vi "AuMT8852B Boolean Attribute.vi"(5 "Value (F)":bool, 7 "Set/Get (Set)":enum16{"Set", "Get"}(ring), 8 "error in (no error)":errorcluster, 10 "Attribute ID":T3, 11 "VISA session":refnum<visa-resource-name>) -> (0 "error out":errorcluster, 3 "VISA session out":refnum<visa-resource-name>, 4 "Value out":bool, 6 "Status":T1=enum."I/O needed")   [LabVIEW 2017]
doc: "Anritsu MT8852B Bluetooth Tester\n\nReconciles attribute values with the cached copies.\n\nINPUTS\nSet/Get - whether the value is being written or read.\nAttribute ID - which value is being written or read.\nValue - attribute to write.\n\nOUTPUTS\nStatus - Instrument I/O will be necessary if simulation is on, caching is off, or caching is on but the cached value is different or invalid.\nValue out - value from the cache."
uses:
  <instrlib>/aumt8852B/General/Utilities/MT8850 Attribute ID.ctl
  <instrlib>/aumt8852B/General/Utilities/Instrument.llb/Instrument Object Reference.ctl
  <instrlib>/aumt8852B/General/Utilities/Instrument.llb/Attribute Status.ctl
panel:
  in  "reference":T2
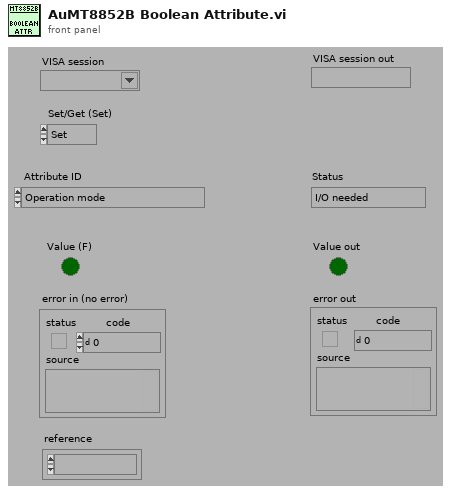
[diagram p1: front panel]
types:
  T1 = typedef "Attribute Status.ctl" = enum16{"No I/O needed", "I/O needed"}
  T2 = typedef "Instrument Object Reference.ctl" = refnum<k1>
  T3 = typedef "MT8850 Attribute ID.ctl" = enum16{"Operation mode", "Selected script", "EUT address source", "EUT Address", "EUT HCI RS232 Baud Rate", "Tester GPIB Address", "Tester RS232 Baud Rate", "Tester Bluetooth Address", "Tester Contrast", "Tester Key Click On", "Tester Modulation Index", "Tester Poll-Null Mode", "Tester Power Range", "Tester RS232 Mode", "Beep on Illegal Entry", "Display User Text", "User Text", "Calibration TX Modulation DAC", "Calibration RX Channel", "Calibration TX Channel", "Calibration TX Power", "Calibration Use TX Table", "Inquiry Request User-friendly Name", "Inquiry Number of Responses", "Inquiry Timeout", "Script Frequency Display", "Script Loop Count", "Script Loop Continuously", "Script Loop Stop on Fail", "Link timeout", "Page timeout", "Filter bandwidth", "SCO air code", "SCO bit position", "SCO input code", "SCO input data", "SCO input sample size", "SCO loopback mode", "SCO packet type", "SCO tone generator", "Tester page scan repetition mode", "Tester follow test mode", "Tester authentication state", "Tester authentication pin code", "Tester authentication pin length"}
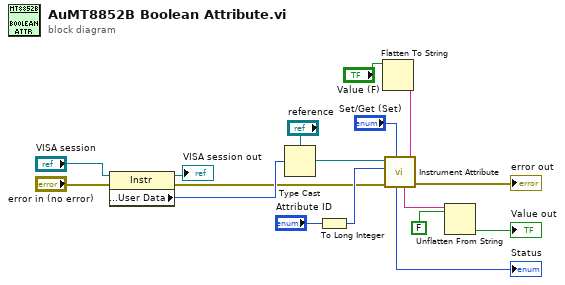
[diagram p0: block diagram]
diagram:
  n1 = property class="Instr"(reference="VISA session", error in="error in (no error)") -> (reference out=→"VISA session out":refnum<visa-resource-name>, error out=w5:errorcluster, "General Settings:User Data"=w11:u32)
  n2 = Type Cast(type="reference", x=w11) -> (*(type *) &x=w9:T2)
  n3 = To Long Integer(number="Attribute ID") -> (32bit integer=w6:i32)
  n4 = Flatten To String(anything="Value (F)") -> (data string=w8:string)  [unwired: 3 in, 2 out]
  n5 = call <instrlib>:"Instrument Attribute.vi"("Flattened value (\"\")"=w8, "Set/Get (Set)"="Set/Get (Set)", "error in (no error)"=w5, "Attribute ID"=w6, "reference"=w9) -> ("error out"=→"error out":errorcluster, "Flattened value out"=w3:string, "I/O needed?"=→"Status":T1)  [unwired: 3 in, 1 out]
  n6 = Unflatten From String(type=FALSE ("Value out"), binary string=w3) -> (value=→"Value out":bool)  [unwired: 3 in, 2 out]
